vi "Scripting_ConvertBaseClassToSubClass.vi"(0 "BaseClass":refnum<vi>, 1 "NewBaseClass":path=path "C:/Documents and Settings/Micke/Skrivbord/My Computer/B_class/B.lvclass", 2 "SubClassTemplate":path=path "C:/Program/National Instruments/LabVIEW 8.2/resource/Framework/Providers/Endevo/ClassProviders/Provider_EndevoGOOP300/Templates/SubTemplate/SubTemplate.lvclass", 3 "GOOP4Style":bool, 5 "error in (no error)":errorcluster) -> (19 "error out":errorcluster={"status"=TRUE, "code"=1055, "source"="Property Node in Scripting_ConvertBaseClassToSubClass.vi"})   [LabVIEW 2012]
uses:
  <vilib>/Utility/miscctls.llb/LVPositionTypeDef.ctl
  <resource>/Framework/Providers/Open_GDS/ClassProviders/Provider_EndevoGOOP300/EndevoProviderName.ctl
  <resource>/Framework/Providers/Open_GDS/ClassProviders/Provider_EndevoGOOP300/Templates/EndevoTemplateNames.ctl
  <resource>/Framework/Providers/Open_GDS/ClassProviders/Provider_EndevoGOOP400/EndevoG4ProviderName.ctl
  <resource>/Framework/Providers/Open_GDS/ClassProviders/Provider_EndevoGOOP400/Templates/EndevoG4TemplateNames.ctl
  <resource>/Framework/Providers/Open_GDS/ClassProviders/Provider_LvNativeClass/ClassWriterNative_class/ClassWriterNative.lvclass
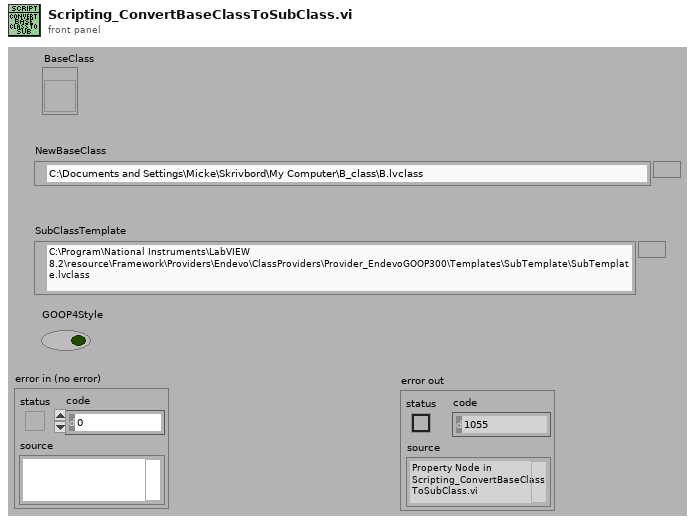
[diagram p1: front panel]
types:
  T1 = cluster{"NewBaseClass":refnum<vi>, "NewBaseCreate ":path, "NewBaseDestroy":path, "NewBaseKernel":path, "NewBaseAttribute":path, "NewBaseClassAttr":path, "NewBaseObjectRef":path, " BaseClass":refnum<vi>, "BaseCreate ":path, "BaseDestroy":path, "BaseKernel":path, "BaseAttribute":path, "BaseClassAttr":path, "BaseClassName":string, "BaseObjectRef":path, "AllBaseClassFiles":path[], "SubNewVi":path, "ObjectRef":refnum<vi>, "BaseNewVi":path, "BaseDeleteVi":path, "SubTemplateKernel":path, "ClassVIs":refnum<vi>[], "SubTemplateClass":refnum<vi>, "BaseTemplateClass":refnum<vi>, "BaseTemplateKernel":path, "BaseAttrRef":refnum<vi>, "BaseClassAttrRef":refnum<vi>, "KernelRef":refnum<vi>, "TemplateVersionUsed":string, "NewBaseNewVI":path, "Singleton":bool, "BaseGetInstance":path, "NewBaseGetInstance":path, "App":refnum<vi>}
  T2 = typedef "LVPositionTypeDef.ctl" = cluster{"Left":i32, "Top":i32}
  T3 = typedef "EndevoTemplateNames.ctl" = enum16{"BaseTemplate", "SubTemplate", "BaseTemplate_4x4x4", "SubTemplate_4x4x4", "SingletonTemplate"}
  T4 = typedef "EndevoProviderName.ctl" = enum16{"EndevoGOOP300"}
  T5 = typedef "EndevoG4TemplateNames.ctl" = enum16{"G4BaseTemplate_Simple_4x4x4", "G4SubTemplate_Simple_4x4x4", "G4BaseTemplate_Simple_6x8x6", "G4SubTemplate_Simple_6x8x6", "G4BaseTemplate_Singleton_4x4x4", "G4SubTemplate_Singleton_4x4x4", "G4BaseTemplate_Singleton_6x8x6", "G4SubTemplate_Singleton_6x8x6", "G4InterfaceTemplate_6x8x6", "G4InterfaceTemplate_4x4x4"}
  T6 = typedef "EndevoG4ProviderName.ctl" = enum16{"EndevoGOOP400"}
  T7 = cluster{"Major":u16, "Minor":u16, "Fix":u16, "Build":u16}
  T8 = cluster{i32, "WireTermSource":refnum<vi>, "AllWireTerminalDrains":refnum<vi>[]}[]
  T9 = cluster{i32, "AllWireTerminalDrains":refnum<vi>[]}[]
  T10 = typedef "GDSLvCLass_ClassSettingsType.ctl" = cluster{"ClassProviderName":string, "ClassTemplateUsed":string, "ClassTemplateVersion":string, "ClassDescription":string, "PlugIns":T11[], "ConnectorPanePattern":string}
  T11 = typedef "GDSLvClass_PlugIn.ctl" = cluster{"Type":T12, "ID":string, "Version":string, "Path":path, "Name":string, "Data":variant}
  T12 = typedef "GDSLvClass_PlugInTypes.ctl" = enum16{"DesignPattern", "MethodTypes"}
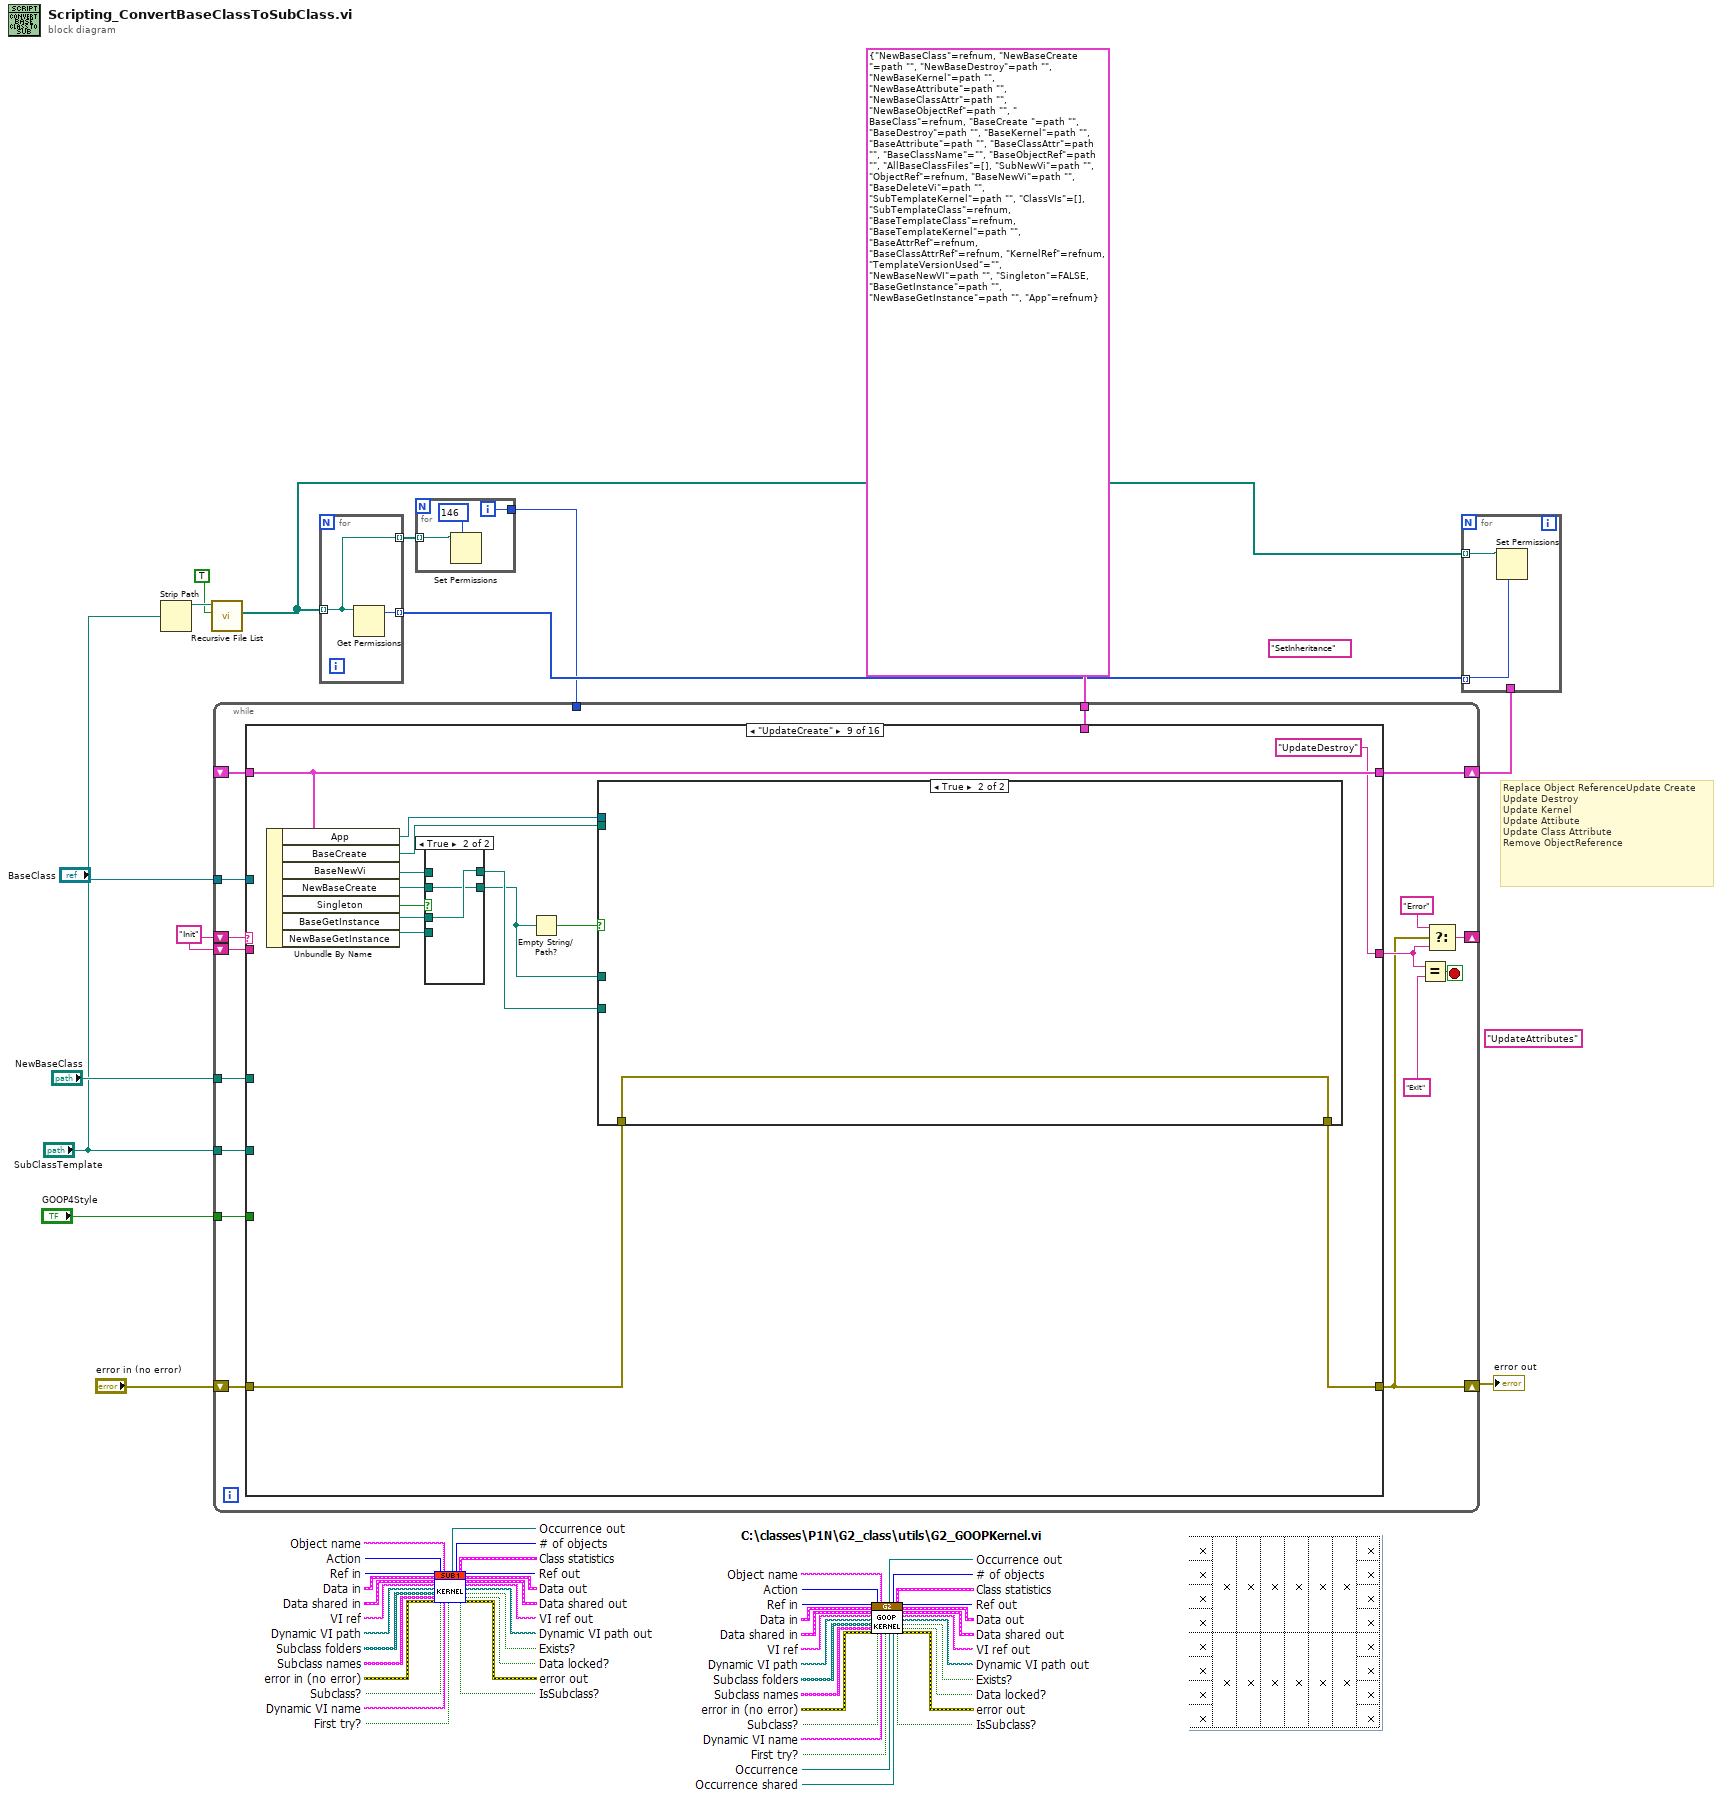
[diagram p0: block diagram]
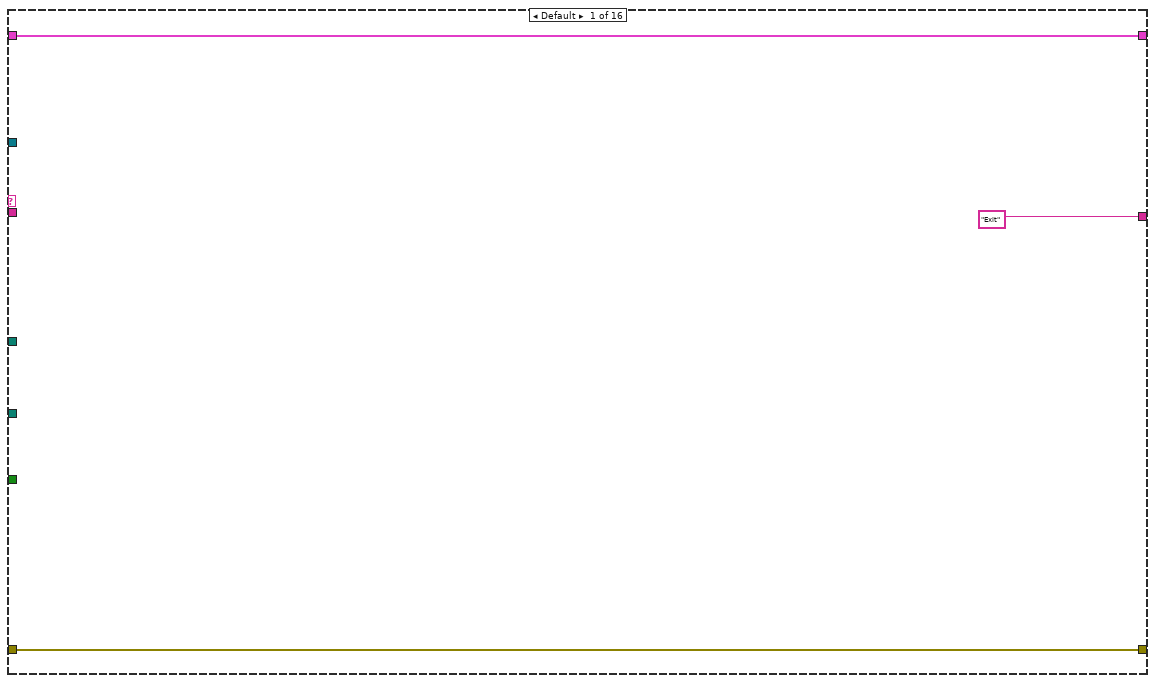
[diagram p2: hidden frame]
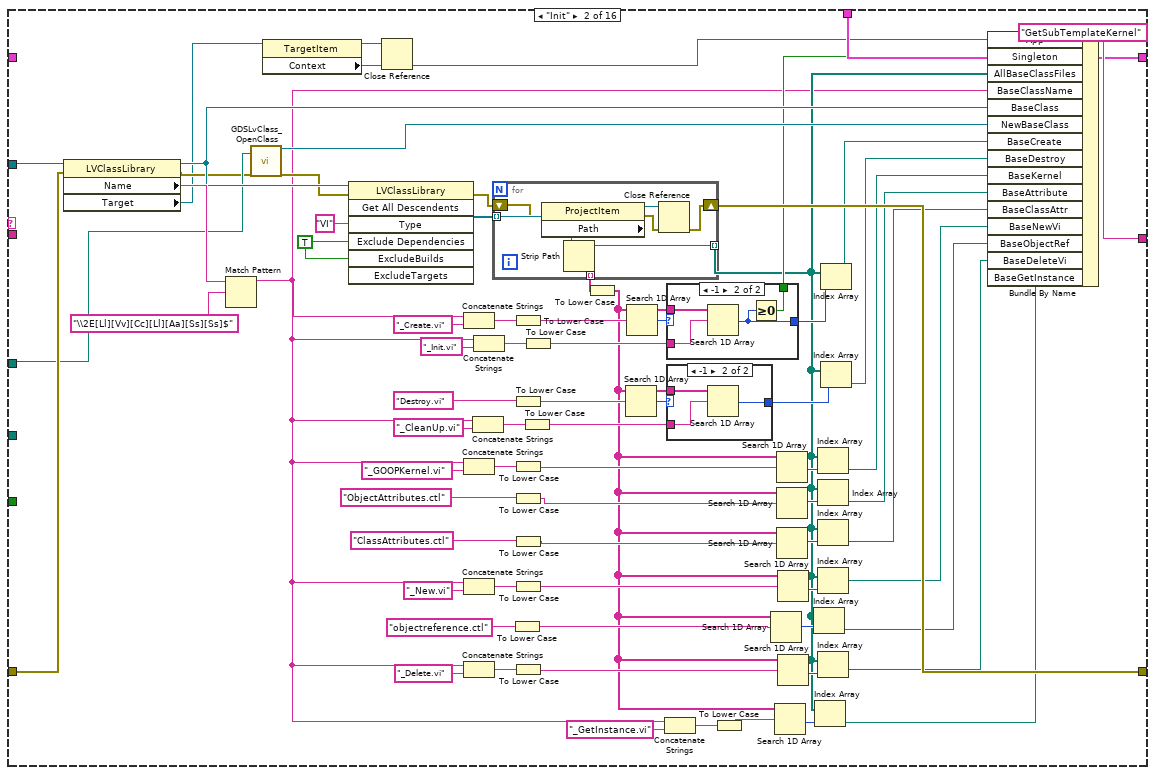
[diagram p3: hidden frame]
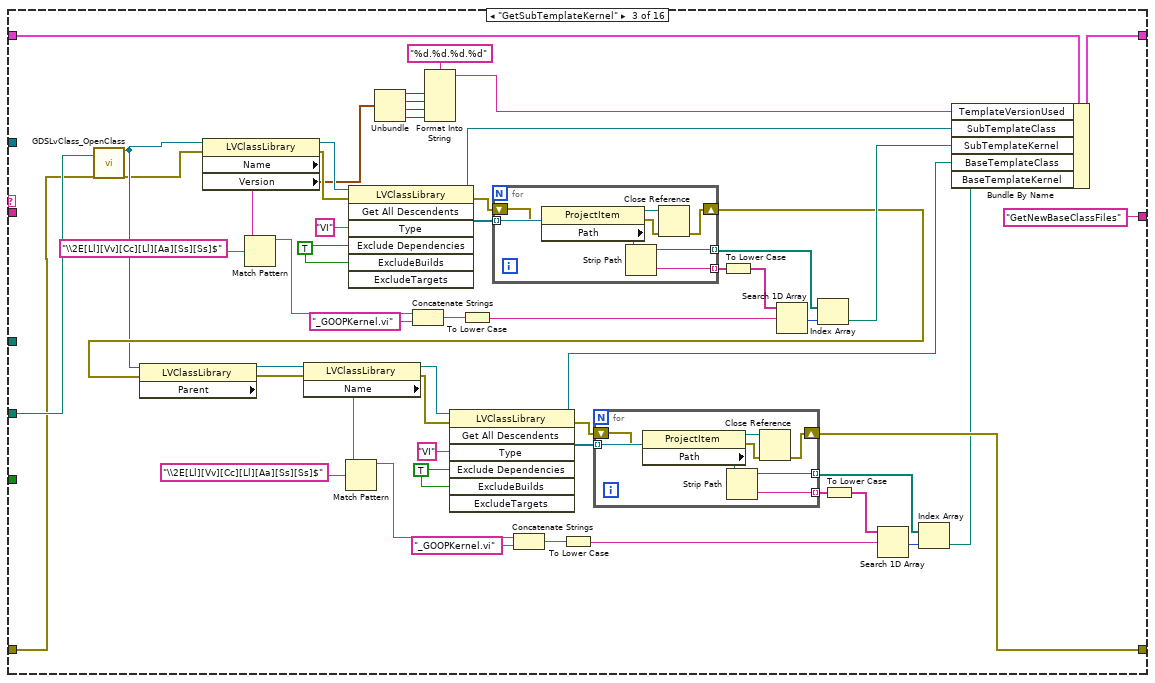
[diagram p6: hidden frame]
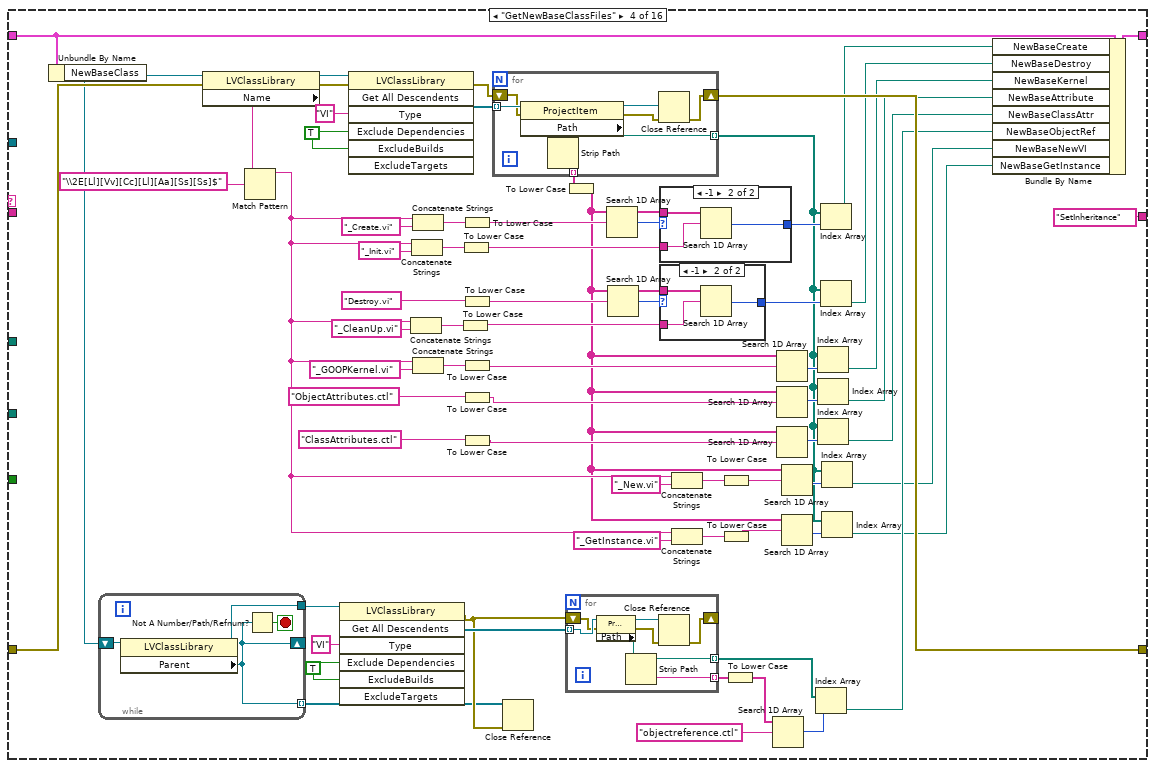
[diagram p7: hidden frame]
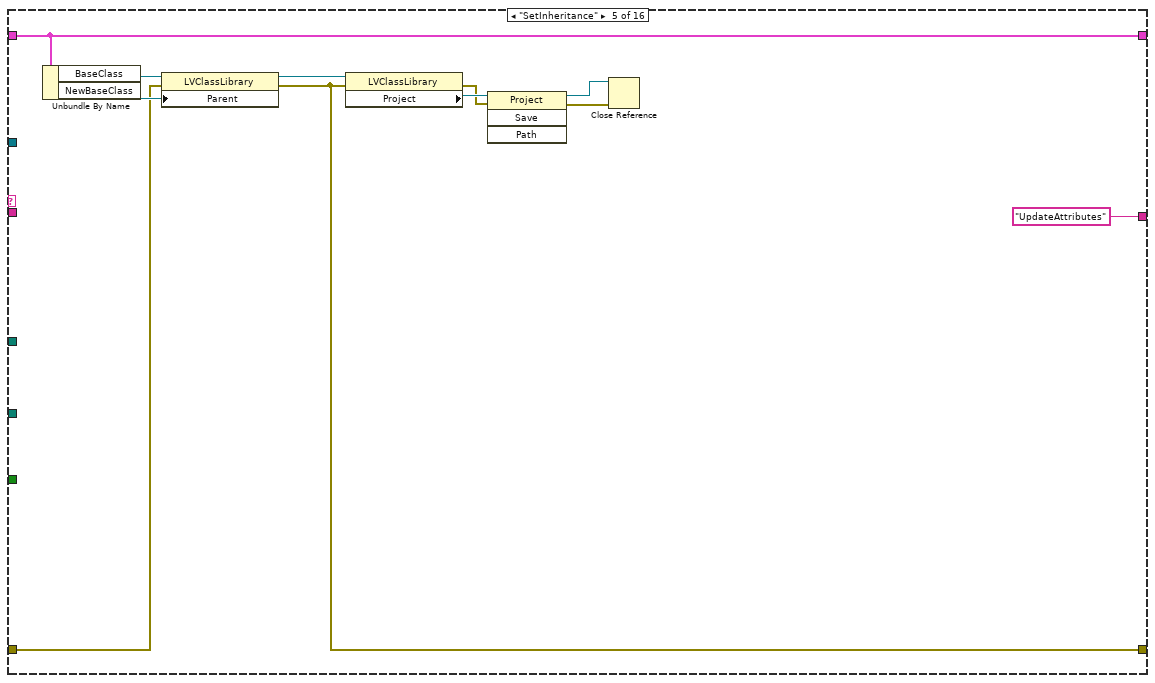
[diagram p10: hidden frame]
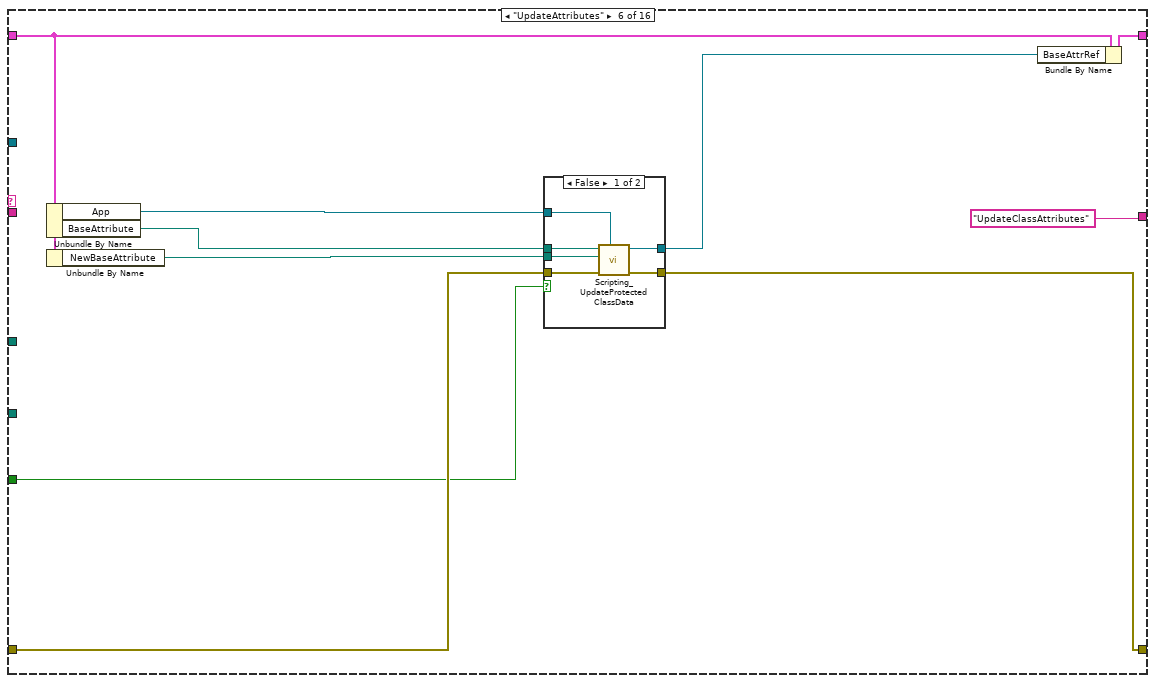
[diagram p11: hidden frame]
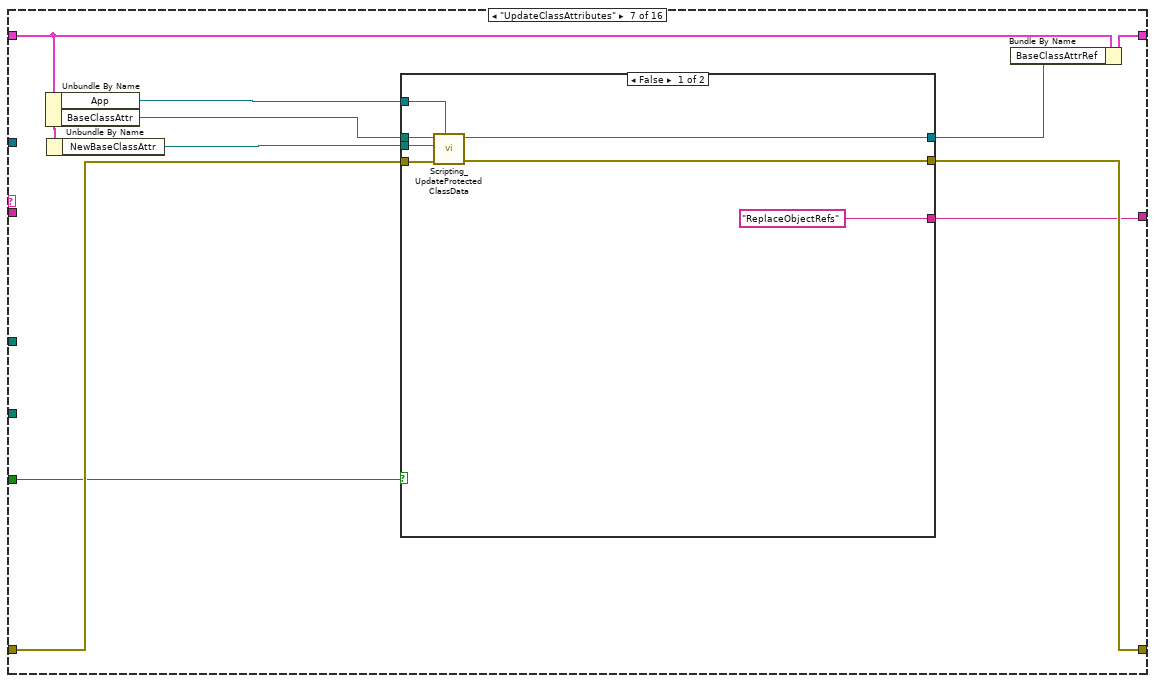
[diagram p13: hidden frame]
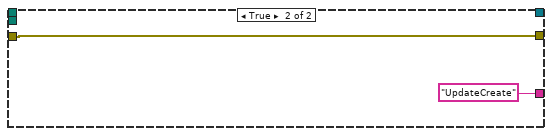
[diagram p14: hidden frame]
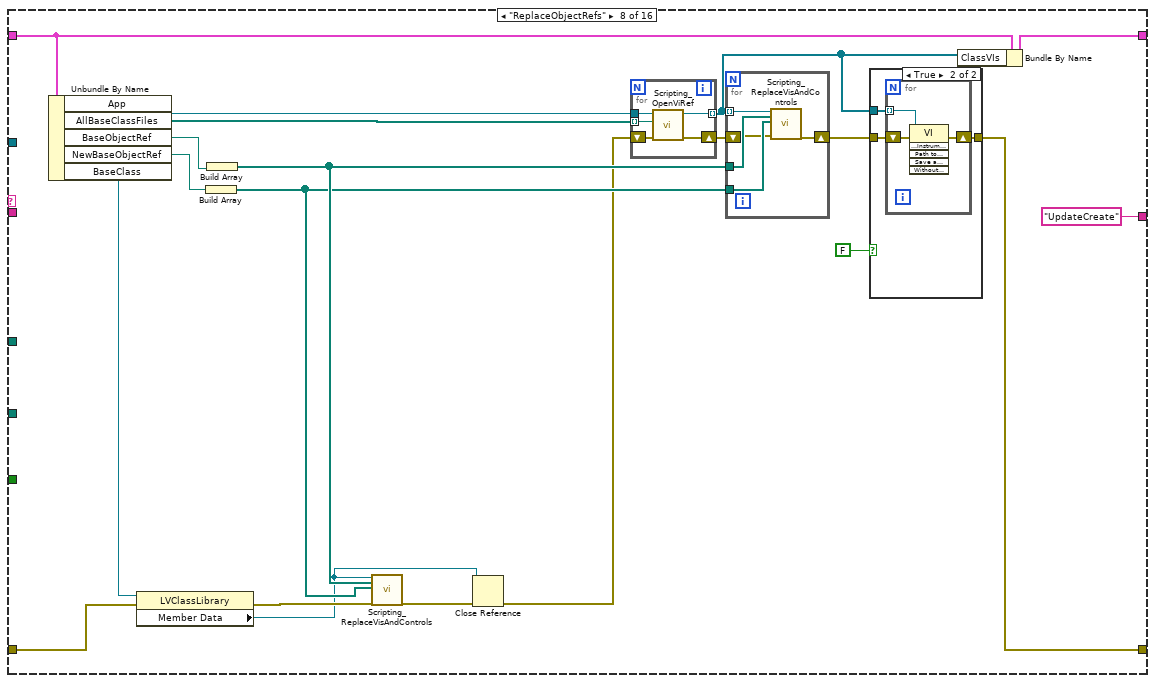
[diagram p15: hidden frame]
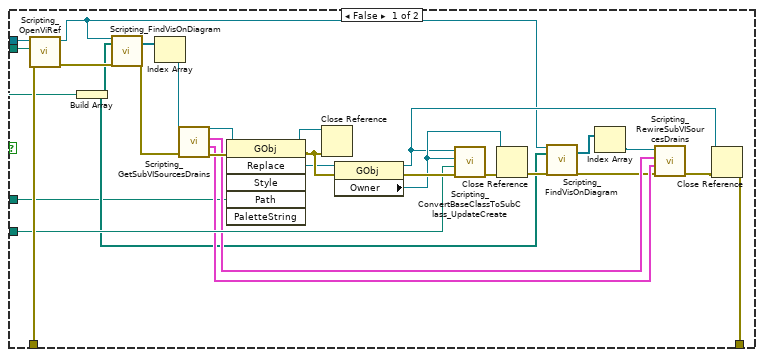
[diagram p17: hidden frame]
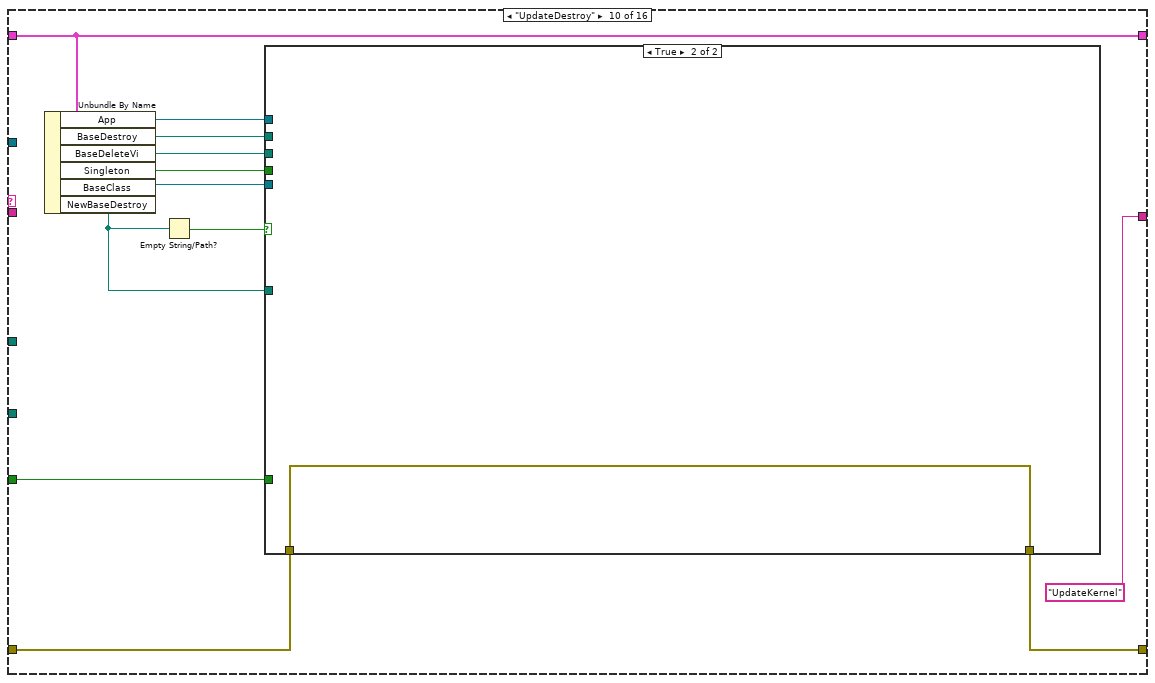
[diagram p19: hidden frame]
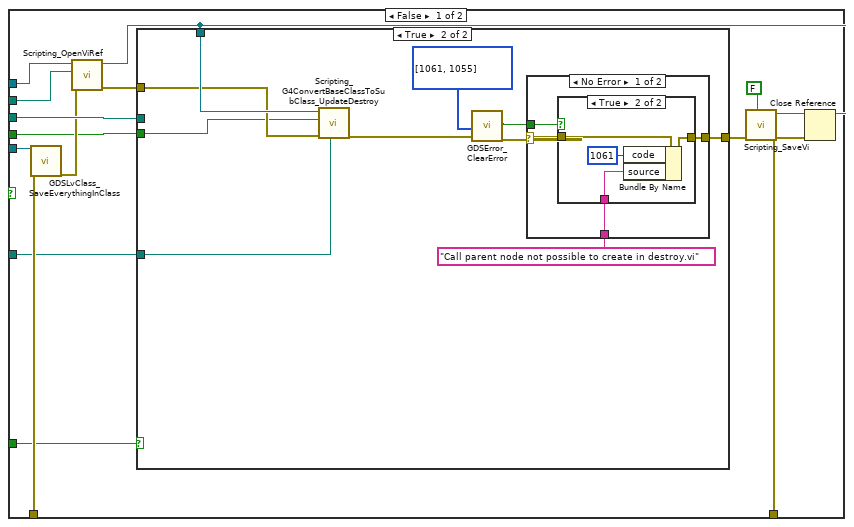
[diagram p20: hidden frame]
diagram:
  (unwired) "SetInheritance"
  (unwired) "UpdateAttributes"
  w10 = "Init"
  # "Replace Object ReferenceUpdate Create\nUpdate Destroy\nUpdate Kernel\nUpdate Attibute\nUpdate Class Attribute\nRemove ObjectReference"
  n1 = Strip Path(path="SubClassTemplate") -> (stripped path=w9:path)  [unwired: 1 out]
  n2 = call <vilib>:"Recursive File List.vi"("Treat LLBs as Folders?"=TRUE, "Folder Path"=w9) -> ("All Files in Dir"=w4:path[])  [unwired: 5 in, 4 out]
  n3 = for {
    tunnel: w4 -> [w16] mode=indexing
    tunnel: [w17] -> w6 mode=indexing
    tunnel: [w16] -> w3 mode=indexing
    n4 = Get Permissions(11:w16) -> (5:w17:i16)  [unwired: 1 in, 4 out]
  }
  n5 = for {
    tunnel: w3 -> [w20] mode=indexing
    tunnel: [w18] -> w5
    i -> [w18]
    n6 = Set Permissions(7:i16 146 ("permissions"), 11:w20) -> ()  [unwired: 3 in, 2 out]
  }
  n7 = while {
    shift-right: [w29] -> w14
    shift-left: "error in (no error)" -> [w36]
    shift-right: [w34] -> _
    shift-left: w10 -> [w35]
    shift-right: [w28] -> w7
    shift-left: _ -> [w27]
    tunnel: "BaseClass" -> [w26]
    tunnel: T1 {"NewBaseClass"=refnum, "NewBaseCreate "=path "", "NewBaseDestroy"=path "", "NewBaseKernel"=path "", "NewBaseAttribute"=path "", "NewBaseClassAttr"=path "", "NewBaseObjectRef"=path "", " BaseClass"=refnum, "BaseCreate "=path "", "BaseDestroy"=path "", "BaseKernel"=path "", "BaseAttribute"=path "", "BaseClassAttr"=path "", "BaseClassName"="", "BaseObjectRef"=path "", "AllBaseClassFiles"=[], "SubNewVi"=path "", "ObjectRef"=refnum, "BaseNewVi"=path "", "BaseDeleteVi"=path "", "SubTemplateKernel"=path "", "ClassVIs"=[], "SubTemplateClass"=refnum, "BaseTemplateClass"=refnum, "BaseTemplateKernel"=path "", "BaseAttrRef"=refnum, "BaseClassAttrRef"=refnum, "KernelRef"=refnum, "TemplateVersionUsed"="", "NewBaseNewVI"=path "", "Singleton"=FALSE, "BaseGetInstance"=path "", "NewBaseGetInstance"=path "", "App"=refnum} -> [w25]
    tunnel: "NewBaseClass" -> [w24]
    tunnel: "SubClassTemplate" -> [w23]
    shift-left: w10 -> [w22]
    tunnel: w5 -> [_]
    tunnel: "GOOP4Style" -> [w21]
    stop <- w33 stop-if-true
    n8 = case shown="\"UpdateCreate\"" w35 {
      tunnel: w36 -> [w39 w79 w139 w238 w301 w312 w327 w349 w389 w431 w505 w645 w675 w717 w762 w772]
      tunnel: [w39 w104 w143 w257 w294 w308 w326 w346 w388 w429 w504 w644 w674 w701 w761 w772] -> w29
      tunnel: ["Exit" "GetSubTemplateKernel" "GetNewBaseClassFiles" "SetInheritance" "UpdateAttributes" "UpdateClassAttributes" w323 "UpdateCreate" "UpdateDestroy" "UpdateKernel" w506 "UpdateClassInfo" "RemoveObjectRef_And_SaveFiles" "UpdateAllDerivedClasses" "CloseReferences" "Exit"] -> w30
      tunnel: [w37 w112 w183 w267 w303 w309 w330 w354 w391 w436 w502 w642 w672 w716 w764 w770] -> w28
      tunnel: w27 -> [w37 _ w171 w239 w303 w310 w331 w355 w391 w436 w503 w642 w672 w716 w764 w770]
      tunnel: w26 -> [_ w78 _ _ _ _ _ _ _ _ _ _ _ _ w760 _]
      tunnel: w25 -> [_ w86 _ _ _ _ _ _ _ _ _ _ _ _ _ _]
      tunnel: w24 -> [_ w66 _ _ _ _ _ _ _ _ _ _ _ _ _ _]
      tunnel: w23 -> [_ _ w168 _ _ _ _ _ _ _ _ _ _ _ _ _]
      tunnel: w22 -> [_ _ _ _ _ _ _ _ _ _ _ _ _ _ _ w771]
      tunnel: w21 -> [_ _ _ _ _ w306 w324 _ _ w430 w501 w646 w665 w699 w759 _]
      frame Default {
      }
      frame "Init" {
        w62 = TRUE ("ExcludeDependencies")
        n9 = property class="LVClassLibrary"(reference=w78, error in=w79) -> (reference out=w76:refnum<vi>, error out=w65:errorcluster, "Name"=w77:string, "Target"=w42:refnum<vi>)
        n10 = Match Pattern(string=w77, regular expression="\\2E[Ll][Vv][Cc][Ll][Aa][Ss][Ss]$") -> (before substring=w44:string)  [unwired: 1 in, 3 out]
        n11 = call <resource>:"GDSLvClass_OpenClass.vi"("ClassToOpen"=w66, "error in (no error)"=w65) -> ("LVClass.Open"=w63:refnum<vi>, "error out"=w64:errorcluster)  [unwired: 16 in]
        n12 = property class="TargetItem"(reference=w42) -> (reference out=w41:refnum<vi>, "Context"=w40:refnum<vi>)  [unwired: 1 in, 1 out]
        n13 = invoke class="LVClassLibrary" method="Get All Descendents"(reference=w76, error in=w64, "Type"="VI", "Exclude Dependencies"=w62, "ExcludeBuilds"=w62) -> (error out=w109:errorcluster, "All Descendents"=w110:refnum<vi>[])  [unwired: 2 in, 5 out]
        n14 = Close Reference(reference=w41) -> ()  [unwired: 1 in, 1 out]
        n15 = Concatenate Strings(w44, "_Create.vi" ("string")) -> (w106:string)
        n16 = Concatenate Strings(w44, "_GOOPKernel.vi" ("string")) -> (w100:string)
        n17 = Concatenate Strings(w44, "_New.vi" ("string")) -> (w83:string)
        n18 = Concatenate Strings(w44, "_Delete.vi" ("string")) -> (w70:string)
        n19 = Concatenate Strings(w44, "_CleanUp.vi" ("string")) -> (w60:string)
        n20 = Concatenate Strings(w44, "_Init.vi" ("string")) -> (w61:string)
        n21 = for {
          tunnel: w110 -> [w129] mode=indexing
          shift-right: [w125] -> w104
          shift-left: w109 -> [w126]
          tunnel: [w124] -> w46 mode=indexing
          tunnel: [w123] -> w107 mode=indexing
          n22 = property class="ProjectItem"(reference=w129, error in=w126) -> (reference out=w128:refnum<vi>, error out=w127:errorcluster, "Path"=w124:path)
          n23 = Strip Path(path=w124) -> (name=w123:string)  [unwired: 1 out]
          n24 = Close Reference(reference=w128, error in (no error)=w127) -> (error out=w125:errorcluster)
        }
        n25 = To Lower Case(string="objectreference.ctl" ("element")) -> (all lower case string=w74:string)
        n26 = To Lower Case(string=w106) -> (all lower case string=w105:string)
        n27 = To Lower Case(string="Destroy.vi") -> (all lower case string=w102:string)
        n28 = To Lower Case(string=w100) -> (all lower case string=w98:string)
        n29 = To Lower Case(string="ObjectAttributes.ctl") -> (all lower case string=w93:string)
        n30 = To Lower Case(string="ClassAttributes.ctl") -> (all lower case string=w90:string)
        n31 = To Lower Case(string=w83) -> (all lower case string=w84:string)
        n32 = To Lower Case(string=w70) -> (all lower case string=w68:string)
        n33 = To Lower Case(string=w60) -> (all lower case string=w58:string)
        n34 = To Lower Case(string=w61) -> (all lower case string=w59:string)
        n35 = To Lower Case(string=w107) -> (all lower case string=w45:string[])
        n36 = Search 1D Array(1D array=w45, element=w102) -> (index of element=w55:i32)  [unwired: 1 in]
        n37 = Search 1D Array(1D array=w45, element=w105) -> (index of element=w57:i32)  [unwired: 1 in]
        n38 = Concatenate Strings(w44, "_GetInstance.vi" ("string")) -> (w49:string)
        n39 = case shown="-1" w57 {
          selector: w57 -> [w118 _]
          tunnel: w45 -> [_ w122]
          tunnel: w59 -> [_ w121]
          tunnel: [w118 w120] -> w56
          tunnel: [_ w119] -> w51
          frame 0, Default {
          }
          frame -1 {
            n40 = Search 1D Array(1D array=w122, element=w121) -> (index of element=w120:i32)  [unwired: 1 in]
            n41 = Greater Or Equal To 0?(x=w120) -> (x >= 0?=w119:bool)
          }
        }
        n42 = case shown="-1" w55 {
          selector: w55 -> [w114 _]
          tunnel: w45 -> [_ w117]
          tunnel: w58 -> [_ w116]
          tunnel: [w114 w115] -> w54
          frame 0, Default {
          }
          frame -1 {
            n43 = Search 1D Array(1D array=w117, element=w116) -> (index of element=w115:i32)  [unwired: 1 in]
          }
        }
        n44 = To Lower Case(string=w49) -> (all lower case string=w47:string)
        n45 = Search 1D Array(1D array=w45, element=w74) -> (index of element=w75:i32)  [unwired: 1 in]
        n46 = Search 1D Array(1D array=w45, element=w47) -> (index of element=w48:i32)  [unwired: 1 in]
        n47 = Search 1D Array(1D array=w45, element=w98) -> (index of element=w97:i32)  [unwired: 1 in]
        n48 = Search 1D Array(1D array=w45, element=w93) -> (index of element=w92:i32)  [unwired: 1 in]
        n49 = Search 1D Array(1D array=w45, element=w90) -> (index of element=w91:i32)  [unwired: 1 in]
        n50 = Search 1D Array(1D array=w45, element=w84) -> (index of element=w81:i32)  [unwired: 1 in]
        n51 = Search 1D Array(1D array=w45, element=w68) -> (index of element=w69:i32)  [unwired: 1 in]
        n52 = Index Array(array=w46, index=w75) -> (element=w72:path)
        n53 = Index Array(array=w46, index=w48) -> (element=w43:path)
        n54 = Index Array(array=w46, index=w97) -> (element=w89:path)
        n55 = Index Array(array=w46, index=w92) -> (element=w88:path)
        n56 = Index Array(array=w46, index=w91) -> (element=w87:path)
        n57 = Index Array(array=w46, index=w81) -> (element=w80:path)
        n58 = Index Array(array=w46, index=w69) -> (element=w67:path)
        n59 = Index Array(array=w46, index=w56) -> (element=w101:path)
        n60 = Index Array(array=w46, index=w54) -> (element=w96:path)
        n61 = Bundle By Name(cluster=w86, "App"=w40, "Singleton"=w51, "AllBaseClassFiles"=w46, "BaseClassName"=w44, "BaseClass"=w76, "NewBaseClass"=w63, "BaseCreate"=w101, "BaseDestroy"=w96, "BaseKernel"=w89, "BaseAttribute"=w88, "BaseClassAttr"=w87, "BaseNewVi"=w80, "BaseObjectRef"=w72, "BaseDeleteVi"=w67, "BaseGetInstance"=w43) -> (w112:T1)
      }
      frame "GetSubTemplateKernel" {
        w137 = TRUE ("ExcludeDependencies")
        w138 = TRUE ("ExcludeDependencies")
        n62 = call <resource>:"GDSLvClass_OpenClass.vi"("ClassToOpen"=w168, "error in (no error)"=w139) -> ("LVClass.Open"=w161:refnum<vi>, "error out"=w140:errorcluster)  [unwired: 16 in]
        n63 = property class="LVClassLibrary"(reference=w161, error in=w140) -> (reference out=w178:refnum<vi>, error out=w179:errorcluster, "Name"=w170:string, "Version"=w131:T7)
        n64 = Match Pattern(string=w170, regular expression="\\2E[Ll][Vv][Cc][Ll][Aa][Ss][Ss]$") -> (before substring=w167:string)  [unwired: 1 in, 3 out]
        n65 = invoke class="LVClassLibrary" method="Get All Descendents"(reference=w178, error in=w179, "Type"="VI", "Exclude Dependencies"=w137, "ExcludeBuilds"=w137) -> (reference out=w163:refnum<vi>, error out=w180:errorcluster, "All Descendents"=w181:refnum<vi>[])  [unwired: 2 in, 4 out]
        n66 = Unbundle(w131) -> ("Major"=w136:u16, "Minor"=w135:u16, "Fix"=w134:u16, "Build"=w133:u16)
        n67 = Concatenate Strings(w167, "_GOOPKernel.vi" ("string")) -> (w176:string)
        n68 = Format Into String(format string="%d.%d.%d.%d", w136, w135, w134, w133) -> (resulting string=w130:string)  [unwired: 2 in, 1 out]
        n69 = To Lower Case(string=w176) -> (all lower case string=w174:string)
        n70 = for {
          tunnel: w181 -> [w197] mode=indexing
          shift-right: [w193] -> w162
          shift-left: w180 -> [w194]
          tunnel: [w192] -> w166 mode=indexing
          tunnel: [w191] -> w177 mode=indexing
          n71 = property class="ProjectItem"(reference=w197, error in=w194) -> (reference out=w196:refnum<vi>, error out=w195:errorcluster, "Path"=w192:path)
          n72 = Strip Path(path=w192) -> (name=w191:string)  [unwired: 1 out]
          n73 = Close Reference(reference=w196, error in (no error)=w195) -> (error out=w193:errorcluster)
        }
        n74 = property class="LVClassLibrary"(reference=w161, error in=w162) -> (error out=w145:errorcluster, "Parent"=w146:refnum<vi>)  [unwired: 1 out]
        n75 = property class="LVClassLibrary"(reference=w146, error in=w145) -> (reference out=w151:refnum<vi>, error out=w150:errorcluster, "Name"=w157:string)
        n76 = Match Pattern(string=w157, regular expression="\\2E[Ll][Vv][Cc][Ll][Aa][Ss][Ss]$") -> (before substring=w158:string)  [unwired: 1 in, 3 out]
        n77 = invoke class="LVClassLibrary" method="Get All Descendents"(reference=w151, error in=w150, "Type"="VI", "Exclude Dependencies"=w138, "ExcludeBuilds"=w138) -> (reference out=w144:refnum<vi>, error out=w149:errorcluster, "All Descendents"=w148:refnum<vi>[])  [unwired: 2 in, 4 out]
        n78 = Concatenate Strings(w158, "_GOOPKernel.vi" ("string")) -> (w153:string)
        n79 = To Lower Case(string=w153) -> (all lower case string=w155:string)
        n80 = for {
          tunnel: w148 -> [w190] mode=indexing
          shift-right: [w186] -> w143
          shift-left: w149 -> [w187]
          tunnel: [w185] -> w159 mode=indexing
          tunnel: [w184] -> w152 mode=indexing
          n81 = property class="ProjectItem"(reference=w190, error in=w187) -> (reference out=w189:refnum<vi>, error out=w188:errorcluster, "Path"=w185:path)
          n82 = Strip Path(path=w185) -> (name=w184:string)  [unwired: 1 out]
          n83 = Close Reference(reference=w189, error in (no error)=w188) -> (error out=w186:errorcluster)
        }
        n84 = To Lower Case(string=w177) -> (all lower case string=w165:string[])
        n85 = Search 1D Array(1D array=w165, element=w174) -> (index of element=w173:i32)  [unwired: 1 in]
        n86 = Index Array(array=w166, index=w173) -> (element=w172:path)
        n87 = To Lower Case(string=w152) -> (all lower case string=w160:string[])
        n88 = Search 1D Array(1D array=w160, element=w155) -> (index of element=w156:i32)  [unwired: 1 in]
        n89 = Index Array(array=w159, index=w156) -> (element=w142:path)
        n90 = Bundle By Name(cluster=w171, "TemplateVersionUsed"=w130, "SubTemplateClass"=w163, "SubTemplateKernel"=w172, "BaseTemplateClass"=w144, "BaseTemplateKernel"=w142) -> (w183:T1)
      }
      frame "GetNewBaseClassFiles" {
        w223 = TRUE ("ExcludeDependencies")
        w224 = TRUE ("ExcludeDependencies")
        n91 = Unbundle By Name(w239) -> ("NewBaseClass"=w236:refnum<vi>)
        n92 = while {
          shift-right: [w284] -> _
          shift-left: w236 -> [w285]
          tunnel: [w284] -> w206 mode=indexing
          tunnel: [w283] -> w234
          stop <- w286 stop-if-true
          n93 = property class="LVClassLibrary"(reference=w285) -> (reference out=w283:refnum<vi>, "Parent"=w284:refnum<vi>)  [unwired: 1 in, 1 out]
          n94 = Not A Number/Path/Refnum?(number/path/refnum=w284) -> (NaN/Path/Refnum?=w286:bool)
        }
        n95 = property class="LVClassLibrary"(reference=w236, error in=w238) -> (reference out=w262:refnum<vi>, error out=w263:errorcluster, "Name"=w237:string)
        n96 = Match Pattern(string=w237, regular expression="\\2E[Ll][Vv][Cc][Ll][Aa][Ss][Ss]$") -> (before substring=w203:string)  [unwired: 1 in, 3 out]
        n97 = invoke class="LVClassLibrary" method="Get All Descendents"(reference=w234, "Type"="VI", "Exclude Dependencies"=w224, "ExcludeBuilds"=w224) -> (error out=w207:errorcluster, "All Descendents"=w233:refnum<vi>[])  [unwired: 3 in, 5 out]
        n98 = invoke class="LVClassLibrary" method="Get All Descendents"(reference=w262, error in=w263, "Type"="VI", "Exclude Dependencies"=w223, "ExcludeBuilds"=w223) -> (error out=w264:errorcluster, "All Descendents"=w265:refnum<vi>[])  [unwired: 2 in, 5 out]
        n99 = Concatenate Strings(w203, "_CleanUp.vi" ("string")) -> (w212:string)
        n100 = Concatenate Strings(w203, "_Init.vi" ("string")) -> (w213:string)
        n101 = Concatenate Strings(w203, "_Create.vi" ("string")) -> (w259:string)
        n102 = Concatenate Strings(w203, "_GOOPKernel.vi" ("string")) -> (w253:string)
        n103 = To Lower Case(string=w212) -> (all lower case string=w208:string)
        n104 = To Lower Case(string=w213) -> (all lower case string=w209:string)
        n105 = To Lower Case(string=w259) -> (all lower case string=w258:string)
        n106 = To Lower Case(string="Destroy.vi") -> (all lower case string=w255:string)
        n107 = To Lower Case(string=w253) -> (all lower case string=w251:string)
        n108 = To Lower Case(string="ObjectAttributes.ctl") -> (all lower case string=w246:string)
        n109 = To Lower Case(string="ClassAttributes.ctl") -> (all lower case string=w243:string)
        n110 = for {
          tunnel: w265 -> [w293] mode=indexing
          shift-right: [w289] -> w257
          shift-left: w264 -> [w290]
          tunnel: [w288] -> w201 mode=indexing
          tunnel: [w287] -> w260 mode=indexing
          n111 = property class="ProjectItem"(reference=w293, error in=w290) -> (reference out=w292:refnum<vi>, error out=w291:errorcluster, "Path"=w288:path)
          n112 = Strip Path(path=w288) -> (name=w287:string)  [unwired: 1 out]
          n113 = Close Reference(reference=w292, error in (no error)=w291) -> (error out=w289:errorcluster)
        }
        n114 = Close Reference(reference=w206, error in (no error)=w207) -> ()  [unwired: 1 out]
        n115 = To Lower Case(string=w260) -> (all lower case string=w200:string[])
        n116 = for {
          tunnel: w233 -> [w282] mode=indexing
          shift-right: [w278] -> _
          shift-left: w207 -> [w279]
          tunnel: [w277] -> w228 mode=indexing
          tunnel: [w276] -> w232 mode=indexing
          n117 = property class="ProjectItem"(reference=w282, error in=w279) -> (reference out=w281:refnum<vi>, error out=w280:errorcluster, "Path"=w277:path)
          n118 = Strip Path(path=w277) -> (name=w276:string)  [unwired: 1 out]
          n119 = Close Reference(reference=w281, error in (no error)=w280) -> (error out=w278:errorcluster)
        }
        n120 = Search 1D Array(1D array=w200, element=w258) -> (index of element=w217:i32)  [unwired: 1 in]
        n121 = Search 1D Array(1D array=w200, element=w255) -> (index of element=w215:i32)  [unwired: 1 in]
        n122 = case shown="-1" w217 {
          selector: w217 -> [w272 _]
          tunnel: w200 -> [_ w275]
          tunnel: w209 -> [_ w274]
          tunnel: [w272 w273] -> w216
          frame 0, Default {
          }
          frame -1 {
            n123 = Search 1D Array(1D array=w275, element=w274) -> (index of element=w273:i32)  [unwired: 1 in]
          }
        }
        n124 = case shown="-1" w215 {
          selector: w215 -> [w268 _]
          tunnel: w200 -> [_ w271]
          tunnel: w208 -> [_ w270]
          tunnel: [w268 w269] -> w214
          frame 0, Default {
          }
          frame -1 {
            n125 = Search 1D Array(1D array=w271, element=w270) -> (index of element=w269:i32)  [unwired: 1 in]
          }
        }
        n126 = Concatenate Strings(w203, "_New.vi" ("string")) -> (w221:string)
        n127 = Concatenate Strings(w203, "_GetInstance.vi" ("string")) -> (w204:string)
        n128 = To Lower Case(string=w221) -> (all lower case string=w222:string)
        n129 = To Lower Case(string=w204) -> (all lower case string=w199:string)
        n130 = To Lower Case(string=w232) -> (all lower case string=w226:string[])
        n131 = Search 1D Array(1D array=w226, element="objectreference.ctl") -> (index of element=w229:i32)  [unwired: 1 in]
        n132 = Search 1D Array(1D array=w200, element=w251) -> (index of element=w250:i32)  [unwired: 1 in]
        n133 = Search 1D Array(1D array=w200, element=w246) -> (index of element=w245:i32)  [unwired: 1 in]
        n134 = Search 1D Array(1D array=w200, element=w243) -> (index of element=w244:i32)  [unwired: 1 in]
        n135 = Search 1D Array(1D array=w200, element=w222) -> (index of element=w219:i32)  [unwired: 1 in]
        n136 = Search 1D Array(1D array=w200, element=w199) -> (index of element=w202:i32)  [unwired: 1 in]
        n137 = Index Array(array=w228, index=w229) -> (element=w227:path)
        n138 = Index Array(array=w201, index=w250) -> (element=w242:path)
        n139 = Index Array(array=w201, index=w245) -> (element=w241:path)
        n140 = Index Array(array=w201, index=w244) -> (element=w240:path)
        n141 = Index Array(array=w201, index=w216) -> (element=w254:path)
        n142 = Index Array(array=w201, index=w214) -> (element=w249:path)
        n143 = Index Array(array=w201, index=w219) -> (element=w218:path)
        n144 = Index Array(array=w201, index=w202) -> (element=w198:path)
        n145 = Bundle By Name(cluster=w239, "NewBaseCreate"=w254, "NewBaseDestroy"=w249, "NewBaseKernel"=w242, "NewBaseAttribute"=w241, "NewBaseClassAttr"=w240, "NewBaseObjectRef"=w227, "NewBaseNewVI"=w218, "NewBaseGetInstance"=w198) -> (w267:T1)
      }
      frame "SetInheritance" {
        n146 = Unbundle By Name(w303) -> ("BaseClass"=w304:refnum<vi>, "NewBaseClass"=w302:refnum<vi>)
        n147 = property class="LVClassLibrary"(reference=w304, error in=w301, "Parent"=w302) -> (reference out=w299:refnum<vi>, error out=w294:errorcluster)
        n148 = property class="LVClassLibrary"(reference=w299, error in=w294) -> (error out=w295:errorcluster, "Project"=w298:refnum<vi>)  [unwired: 1 out]
        n149 = invoke class="Project" method="Save"(reference=w298, error in=w295) -> (reference out=w296:refnum<vi>, error out=w297:errorcluster)  [unwired: 2 in, 2 out]
        n150 = Close Reference(reference=w296, error in (no error)=w297) -> ()  [unwired: 1 out]
      }
      frame "UpdateAttributes" {
        n151 = Unbundle By Name(w310) -> ("App"=w305:refnum<vi>, "BaseAttribute"=w313:path)
        n152 = Unbundle By Name(w310) -> ("NewBaseAttribute"=w311:path)
        n153 = case shown="False" w306 {
          tunnel: w313 -> [w320 _]
          tunnel: w312 -> [w319 w321]
          tunnel: w311 -> [w318 _]
          tunnel: [w317 w321] -> w308
          tunnel: [w316 _] -> w307
          tunnel: w305 -> [w315 _]
          frame False {
            n154 = call <resource>:"Scripting_UpdateProtectedClassData.vi"("AppRef"=w315, "error in (no error)"=w319, "NewBaseAttribute"=w318, "BaseAttribute"=w320) -> ("error out"=w317:errorcluster, "BaseAttributeReference"=w316:refnum<vi>)  [unwired: 6 in]
          }
          frame True {
          }
        }
        n155 = Bundle By Name(cluster=w310, "BaseAttrRef"=w307) -> (w309:T1)
      }
      frame "UpdateClassAttributes" {
        n156 = Unbundle By Name(w331) -> ("App"=w322:refnum<vi>, "BaseClassAttr"=w329:path)
        n157 = Unbundle By Name(w331) -> ("NewBaseClassAttr"=w328:path)
        n158 = case shown="False" w324 {
          tunnel: w329 -> [w338 _]
          tunnel: w328 -> [w337 _]
          tunnel: w327 -> [w336 w340]
          tunnel: [w335 w340] -> w326
          tunnel: [w334 _] -> w325
          tunnel: ["ReplaceObjectRefs" "UpdateCreate"] -> w323
          tunnel: w322 -> [w332 _]
          frame False {
            n159 = call <resource>:"Scripting_UpdateProtectedClassData.vi"("AppRef"=w332, "error in (no error)"=w336, "NewBaseAttribute"=w337, "BaseAttribute"=w338) -> ("error out"=w335:errorcluster, "BaseAttributeReference"=w334:refnum<vi>)  [unwired: 6 in]
          }
          frame True {
          }
        }
        n160 = Bundle By Name(cluster=w331, "BaseClassAttrRef"=w325) -> (w330:T1)
      }
      frame "ReplaceObjectRefs" {
        n161 = Unbundle By Name(w355) -> ("App"=w341:refnum<vi>, "AllBaseClassFiles"=w352:path[], "BaseObjectRef"=w359:path, "NewBaseObjectRef"=w358:path, "BaseClass"=w350:refnum<vi>)
        n162 = property class="LVClassLibrary"(reference=w350, error in=w349) -> (error out=w348:errorcluster, "Member Data"=w345:refnum<vi>)  [unwired: 1 out]
        n163 = Build Array(w358) -> (w356:path[])
        n164 = Build Array(w359) -> (w357:path[])
        n165 = call <resource>:"Scripting_ReplaceVisAndControls.vi"("ViRef"=w345, "OldVIsAndControls"=w357, "NewVIsAndControls"=w356, "error in (no error)"=w348) -> ("error out"=w342:errorcluster)  [unwired: 14 in, 1 out]
        n166 = Close Reference(reference=w345, error in (no error)=w342) -> (error out=w347:errorcluster)
        n167 = for {
          shift-right: [w372] -> w344
          shift-left: w347 -> [w371]
          tunnel: w352 -> [w370] mode=indexing
          tunnel: [w369] -> w351 mode=indexing
          tunnel: w341 -> [w368]
          n168 = call <resource>:"Scripting_OpenViRef.vi"("error in"=w371, "ViPath/ViName"=w370, "AppRef"=w368) -> ("error out"=w372:errorcluster, "vi reference"=w369:refnum<vi>)  [unwired: 7 in]
        }
        n169 = for {
          shift-right: [w377] -> w353
          shift-left: w344 -> [w374]
          tunnel: w357 -> [w376]
          tunnel: w356 -> [w375]
          tunnel: w351 -> [w373] mode=indexing
          n170 = call <resource>:"Scripting_ReplaceVisAndControls.vi"("ViRef"=w373, "OldVIsAndControls"=w376, "NewVIsAndControls"=w375, "error in (no error)"=w374) -> ("error out"=w377:errorcluster)  [unwired: 14 in, 1 out]
        }
        n171 = case shown="True" FALSE {
          tunnel: w353 -> [w361 w364]
          tunnel: w351 -> [_ w363]
          tunnel: [w361 w362] -> w346
          frame False {
          }
          frame True {
            n172 = for {
              shift-right: [w366] -> w362
              shift-left: w364 -> [w367]
              tunnel: w363 -> [w365] mode=indexing
              n173 = invoke class="VI" method="Save.Instrument"(reference=w365, error in=w367) -> (error out=w366:errorcluster)  [unwired: 4 in, 5 out]
            }
          }
        }
        n174 = Bundle By Name(cluster=w355, "ClassVIs"=w351) -> (w354:T1)
      }
      frame "UpdateCreate" {
        n175 = Unbundle By Name(w391) -> ("App"=w381:refnum<vi>, "BaseCreate"=w390:path, "BaseNewVi"=w386:path, "NewBaseCreate"=w385:path, "Singleton"=w387:bool, "BaseGetInstance"=w383:path, "NewBaseGetInstance"=w382:path)
        n176 = case shown="True" w387 {
          tunnel: w386 -> [w422 _]
          tunnel: w385 -> [w421 w423]
          tunnel: [w422 w424] -> w384
          tunnel: [w421 w423] -> w380
          tunnel: w383 -> [_ w424]
          tunnel: w382 -> [_ _]
          frame False {
          }
          frame True {
          }
        }
        n177 = Empty String/Path?(string/path=w380) -> (empty?=w378:bool)
        n178 = case shown="True" w378 {
          tunnel: w390 -> [w419 _]
          tunnel: w389 -> [w418 w420]
          tunnel: [w409 w420] -> w388
          tunnel: w384 -> [w408 _]
          tunnel: w381 -> [w393 _]
          tunnel: w380 -> [w392 _]
          frame False {
            n179 = call <resource>:"Scripting_OpenViRef.vi"("error in"=w418, "ViPath/ViName"=w419, "AppRef"=w393) -> ("error out"=w417:errorcluster, "vi reference"=w398:refnum<vi>)  [unwired: 7 in]
            n180 = Build Array(w408) -> (w397:path[])
            n181 = call <resource>:"Scripting_FindVisOnDiagram.vi"("ViRef"=w398, "VIsToSerachFor/ViName"=w397, "error in (no error)"=w417) -> ("VisFound"=w416:refnum<vi>[], "error out"=w407:errorcluster)  [unwired: 15 in]
            n182 = Index Array(array=w416) -> (element=w406:refnum<vi>)  [unwired: 1 in]
            n183 = call <resource>:"Scripting_GetSubVISourcesDrains.vi"("error in (no error)"=w407, "SubVIIn"=w406) -> ("error out"=w405:errorcluster, "DrainsSources"=w401:T8, "SourceDrains"=w402:T9, "SubVIOut"=w404:refnum<vi>)  [unwired: 6 in]
            n184 = invoke class="GObj" method="Replace"(reference=w404, error in=w405, "Path"=w392) -> (reference out=w415:refnum<vi>, error out=w414:errorcluster, "Replace"=w413:refnum<vi>)  [unwired: 3 in, 3 out]
            n185 = Close Reference(reference=w415, error in (no error)=w414) -> ()  [unwired: 1 out]
            n186 = property class="GObj"(reference=w413, error in=w414) -> (reference out=w400:refnum<vi>, error out=w412:errorcluster, "Owner"=w411:refnum<vi>)
            n187 = call <resource>:"Scripting_ConvertBaseClassToSubClass_UpdateCreate.vi"("error in (no error)"=w412, "NewViPath"=w408, "Diagram"=w411, "NewBaseCreate"=w400) -> ("error out"=w410:errorcluster)  [unwired: 7 in]
            n188 = Close Reference(reference=w411, error in (no error)=w410) -> (error out=w399:errorcluster)
            n189 = call <resource>:"Scripting_FindVisOnDiagram.vi"("ViRef"=w398, "VIsToSerachFor/ViName"=w397, "error in (no error)"=w399) -> ("VisFound"=w394:refnum<vi>[], "error out"=w395:errorcluster)  [unwired: 15 in]
            n190 = Index Array(array=w394) -> (element=w396:refnum<vi>)  [unwired: 1 in]
            n191 = call <resource>:"Scripting_RewireSubVISourcesDrains.vi"("error in"=w395, "DrainsSources"=w401, "SourceDrains"=w402, "SubVIIn"=w396) -> ("error out"=w403:errorcluster)  [unwired: 7 in]
            n192 = Close Reference(reference=w400, error in (no error)=w403) -> (error out=w409:errorcluster)
          }
          frame True {
          }
        }
      }
      frame "UpdateDestroy" {
        n193 = Unbundle By Name(w436) -> ("App"=w427:refnum<vi>, "BaseDestroy"=w435:path, "BaseDeleteVi"=w434:path, "Singleton"=w428:bool, "BaseClass"=w432:refnum<vi>, "NewBaseDestroy"=w426:path)
        n194 = Empty String/Path?(string/path=w426) -> (empty?=w425:bool)
        n195 = case shown="True" w425 {
          tunnel: w435 -> [w451 _]
          tunnel: w434 -> [w449 _]
          tunnel: w432 -> [w446 _]
          tunnel: w431 -> [w445 w500]
          tunnel: w430 -> [w442 _]
          tunnel: [w441 w500] -> w429
          tunnel: w428 -> [w439 _]
          tunnel: w427 -> [w438 _]
          tunnel: w426 -> [w437 _]
          frame False {
            n196 = call <resource>:"GDSLvClass_SaveEverythingInClass.vi"("ClassRefIn"=w446, "error in"=w445) -> ("error out"=w443:errorcluster)  [unwired: 16 in, 1 out]
            n197 = call <resource>:"Scripting_OpenViRef.vi"("error in"=w443, "ViPath/ViName"=w451, "AppRef"=w438) -> ("error out"=w450:errorcluster, "vi reference"=w447:refnum<vi>)  [unwired: 7 in]
            n198 = case shown="True" w442 {
              tunnel: w450 -> [w469 w482]
              tunnel: w449 -> [w464 _]
              tunnel: w447 -> [w460 w483]
              tunnel: [w454 w485] -> w444
              tunnel: w437 -> [w453 w484]
              tunnel: w439 -> [_ w480]
              frame False {
                n199 = Build Array(w464) -> (w468:path[])
                n200 = call <resource>:"Scripting_FindVisOnDiagram.vi"("ViRef"=w460, "VIsToSerachFor/ViName"=w468, "error in (no error)"=w469) -> ("VisFound"=w467:refnum<vi>[], "error out"=w463:errorcluster)  [unwired: 15 in]
                n201 = Index Array(array=w467) -> (element=w461:refnum<vi>)  [unwired: 1 in]
                n202 = property class="GObj"(reference=w461, error in=w463) -> (reference out=w466:refnum<vi>, error out=w465:errorcluster, "Owner"=w452:refnum<vi>)
                n203 = call <resource>:"Scripting_ConvertBaseClassToSubClass_UpdateDestroy.vi"("BaseClassDestroyViPath"=w453, "error in (no error)"=w465, "Diagram"=w452, "DeleteViRef"=w466) -> ("error out"=w462:errorcluster)  [unwired: 7 in]
                n204 = Close Reference(reference=w452, error in (no error)=w462) -> (error out=w459:errorcluster)
                n205 = call <resource>:"GDSError_ClearError.vi"("codes"=i32[] [1061, 1055], "error in (no error)"=w459) -> ("Cleared?"=w456:bool, "error out"=w457:errorcluster)  [unwired: 16 in]
                n206 = case shown="No Error" w457 {
                  selector: w457 -> [w472 w479]
                  tunnel: w456 -> [w473 _]
                  tunnel: "Call parent node not possible to create in destroy.vi" ("source") -> [w471 _]
                  tunnel: [w470 w479] -> w454
                  frame No Error {
                    n207 = case shown="True" w473 {
                      tunnel: w472 -> [w474 w478]
                      tunnel: w471 -> [_ w476]
                      tunnel: [w474 w475] -> w470
                      frame False {
                      }
                      frame True {
                        n208 = Bundle By Name(cluster=w478, "code"=1061, "source"=w476) -> (w475:errorcluster)
                      }
                    }
                  }
                  frame Error {
                  }
                }
              }
              frame True {
                n209 = call <resource>:"Scripting_G4ConvertBaseClassToSubClass_UpdateDestroy.vi"("BaseClassDestroyViPath"=w484, "error in (no error)"=w482, "Singleton"=w480, "ViRef"=w483) -> ("error out"=w481:errorcluster)  [unwired: 7 in]
                n210 = call <resource>:"GDSError_ClearError.vi"("codes"=i32[] [1061, 1055], "error in (no error)"=w481) -> ("Cleared?"=w487:bool, "error out"=w488:errorcluster)  [unwired: 16 in]
                n211 = case shown="No Error" w488 {
                  selector: w488 -> [w492 w499]
                  tunnel: w487 -> [w493 _]
                  tunnel: "Call parent node not possible to create in destroy.vi" ("source") -> [w491 _]
                  tunnel: [w490 w499] -> w485
                  frame No Error {
                    n212 = case shown="True" w493 {
                      tunnel: w492 -> [w494 w498]
                      tunnel: w491 -> [_ w496]
                      tunnel: [w494 w495] -> w490
                      frame False {
                      }
                      frame True {
                        n213 = Bundle By Name(cluster=w498, "code"=1061, "source"=w496) -> (w495:errorcluster)
                      }
                    }
                  }
                  frame Error {
                  }
                }
              }
            }
            n214 = call <resource>:"Scripting_SaveVi.vi"("ForceResaving(False)"=FALSE, "error in (no error)"=w444, "VIRefToSaveIn"=w447) -> ("error out"=w441:errorcluster, "VIRefToSaveOut"=w440:refnum<vi>)  [unwired: 7 in]
            n215 = Close Reference(reference=w440, error in (no error)=w441) -> ()  [unwired: 1 out]
          }
          frame True {
          }
        }
      }
      frame "UpdateKernel" {
        n216 = case shown="False" w501 {
          tunnel: ["UpdateClassInfo" "UpdateNEWVI"] -> w506
          tunnel: w505 -> [w560 w626]
          tunnel: [w512 w627] -> w504
          tunnel: w503 -> [w508 w625]
          tunnel: [w530 w624] -> w502
          frame False {
            n217 = Unbundle By Name(w508) -> ("App"=w507:refnum<vi>, "BaseKernel"=w581:path, "SubTemplateKernel"=w527:path)
            n218 = call <resource>:"Scripting_OpenViRef.vi"("error in"=w560, "ViPath/ViName"=w581, "AppRef"=w507) -> ("error out"=w580:errorcluster, "vi reference"=w571:refnum<vi>)  [unwired: 7 in]
            n219 = property class="VI"(reference=w571, error in=w580) -> (reference out=w566:refnum<vi>, error out=w529:errorcluster, "Diagram"=w569:refnum<vi>)
            n220 = Unbundle By Name(w508) -> ("SubTemplateClass"=w515:refnum<vi>, "BaseClass"=w514:refnum<vi>)
            n221 = property class="TopLvlDiag"(reference=w569, error in=w529) -> (reference out=w563:refnum<vi>, error out=w568:errorcluster, "AllObjs[]"=w567:refnum<vi>[])
            n222 = Unbundle By Name(w508) -> ("BaseAttribute"=w548:path, "BaseClassAttr"=w543:path, "BaseTemplateKernel"=w535:path, "NewBaseKernel"=w533:path)
            n223 = for {
              tunnel: w568 -> [w616]
              tunnel: w567 -> [w617] mode=indexing
              tunnel: [w616] -> w565
              n224 = invoke class="GObj" method="Delete"(reference=w617, error in=w616) -> (reference out=w618:refnum<vi>)  [unwired: 1 in, 2 out]
              n225 = Close Reference(reference=w618) -> ()  [unwired: 1 in, 1 out]
            }
            n226 = invoke class="VI" method="BD.Remove Bad Wires"(reference=w566, error in=w565) -> (reference out=w562:refnum<vi>, error out=w528:errorcluster)  [unwired: 1 in, 1 out]
            n227 = call <resource>:"Scripting_OpenViRef.vi"("error in"=w528, "ViPath/ViName"=w527, "AppRef"=w507) -> ("error out"=w525:errorcluster, "vi reference"=w524:refnum<vi>)  [unwired: 7 in]
            n228 = invoke class="VI" method="Fake Exec State"(reference=w524, "state"=2 ("State")) -> (reference out=w523:refnum<vi>)  [unwired: 2 in, 3 out]
            n229 = property class="VI"(reference=w523, error in=w525) -> (reference out=w520:refnum<vi>, error out=w579:errorcluster, "Diagram"=w576:refnum<vi>)
            n230 = invoke class="TopLvlDiag" method="Select All"(reference=w576, error in=w579) -> (reference out=w577:refnum<vi>, error out=w578:errorcluster)  [unwired: 1 in, 1 out]
            n231 = invoke class="TopLvlDiag" method="Copy Selection"(reference=w577, error in=w578) -> (reference out=w521:refnum<vi>, error out=w564:errorcluster)  [unwired: 1 in, 1 out]
            n232 = invoke class="TopLvlDiag" method="Paste"(reference=w563, error in=w564, "Pos"=T2 {"Left"=50, "Top"=50} ("Position")) -> (reference out=w541:refnum<vi>, error out=w542:errorcluster)  [unwired: 1 in, 2 out]
            n233 = invoke class="App" method="Clipboard.Empty"(error in=w542) -> (error out=w522:errorcluster)  [unwired: 2 in, 2 out]
            n234 = property class="VI"(reference=w562, error in=w522) -> (error out=w573:errorcluster, "Panel"=w574:refnum<vi>)  [unwired: 1 out]
            n235 = Close Reference(reference=w541) -> ()  [unwired: 1 in, 1 out]
            n236 = property class="Pnl"(reference=w574, error in=w573) -> (reference out=w540:refnum<vi>, error out=w572:errorcluster, "Controls[]"=w538:refnum<vi>[])
            n237 = Build Array(w533) -> (w532:path[])
            n238 = Build Array(w535) -> (w534:path[])
            n239 = Close Reference(reference=w521, error in (no error)=w522) -> (error out=w539:errorcluster)
            n240 = Close Reference(reference=w520, error in (no error)=w539) -> ()  [unwired: 1 out]
            n241 = for {
              tunnel: w538 -> [w619] mode=indexing
              shift-right: [w621] -> w570
              shift-left: w572 -> [w622]
              tunnel: [w620] -> w516 mode=indexing
              n242 = property class="Ctl"(reference=w619, error in=w622) -> (error out=w621:errorcluster, "Label.Text"=w620:string)  [unwired: 1 out]
            }
            n243 = property class="VI"(reference=w571, error in=w570) -> (reference out=w509:refnum<vi>, error out=w561:errorcluster, "ConPane"=w536:refnum<vi>)
            n244 = Search 1D Array(1D array=w516, element="Dynamic VI path" ("Id")) -> (index of element=w510:i32)  [unwired: 1 in]
            n245 = case shown="Default" w510 {
              tunnel: [string[] ["Data in", "Data out", "Action", "Ref in", "Ref out", "Data locked?", "error out", "error in (no error)", "Subclass?", "Object name", "Exists?", "Data shared out", "Data shared in", "Subclass names", "Class name", "Probe in", "Class statistics", "IsSubclass?", "Misc", "# of objects", "Occurrence out", "Occurrence", "Occurrence shared", "Probe out"] ("Array") string[] ["Data in", "Data out", "Action", "Ref in", "Ref out", "Data locked?", "error out", "error in (no error)", "Subclass?", "Object name", "Exists?", "Data shared out", "Data shared in", "Subclass folders", "Subclass names", "Dynamic VI name", "VI ref out", "Dynamic VI path", "Dynamic VI path out", "VI ref", "Class statistics", "IsSubclass?", "First try?", "# of objects", "Occurrence out", "Occurrence", "Occurrence shared"] ("Array")] -> w519
              tunnel: [i32[] [1, 21, 8, 0, 20, 26, 27, 7, 9, 10, 25, 22, 2, 6, 11, 3, 18, 19, 13, 16, 14, 15, 17, 23] i32[] [1, 21, 8, 0, 20, 26, 27, 7, 9, 10, 25, 22, 2, 5, 6, 11, 23, 4, 24, 3, 18, 19, 13, 16, 14, 15, 17]] -> w518
              frame -1 {
              }
              frame Default {
              }
            }
            n246 = for {
              tunnel: w516 -> [w606] mode=indexing
              tunnel: w536 -> [w615]
              tunnel: w519 -> [w608]
              tunnel: w538 -> [w609] mode=indexing
              tunnel: w518 -> [w613]
              shift-right: [w610] -> w537
              shift-left: w561 -> [w611]
              n247 = Search and Replace String(replace all?=TRUE ("replace all? (F)"), input string=w606, search string="\n", replace string=" " ("replace string (\"\")")) -> (result string=w605:string)  [unwired: 4 in, 3 out]
              n248 = Search 1D Array(1D array=w608, element=w605) -> (index of element=w614:i32)  [unwired: 1 in]
              n249 = Index Array(array=w613, index=w614) -> (element=w612:i32)
              n250 = invoke class="ConPane" method="AssignCtrlToTerm"(reference=w615, error in=w611, "Control"=w609, "TermIdx"=w612) -> (error out=w610:errorcluster)  [unwired: 1 in, 4 out]
            }
            n251 = Close Reference(reference=w536, error in (no error)=w537) -> ()  [unwired: 1 out]
            n252 = Search 1D Array(1D array=w516, element="Data in" ("Label.Text")) -> (index of element=w559:i32)  [unwired: 1 in]
            n253 = Search 1D Array(1D array=w516, element="Data out" ("Label.Text")) -> (index of element=w555:i32)  [unwired: 1 in]
            n254 = Search 1D Array(1D array=w516, element="Data shared in" ("Label.Text")) -> (index of element=w554:i32)  [unwired: 1 in]
            n255 = Search 1D Array(1D array=w516, element="Data shared out" ("Label.Text")) -> (index of element=w553:i32)  [unwired: 1 in]
            n256 = Index Array(array=w538, index=w559) -> (element=w557:refnum<vi>)
            n257 = Index Array(array=w538, index=w555) -> (element=w549:refnum<vi>)
            n258 = Index Array(array=w538, index=w554) -> (element=w545:refnum<vi>)
            n259 = Index Array(array=w538, index=w553) -> (element=w544:refnum<vi>)
            n260 = invoke class="Ctl" method="Replace"(reference=w557, error in=w537, "Path"=w548) -> (error out=w556:errorcluster)  [unwired: 3 in, 5 out]
            n261 = invoke class="Ctl" method="Replace"(reference=w549, error in=w556, "Path"=w548) -> (error out=w546:errorcluster)  [unwired: 3 in, 5 out]
            n262 = Close Reference(reference=w540) -> ()  [unwired: 1 in, 1 out]
            n263 = invoke class="Ctl" method="Replace"(reference=w545, error in=w546, "Path"=w543) -> (error out=w547:errorcluster)  [unwired: 3 in, 5 out]
            n264 = Bundle By Name(cluster=w508, "KernelRef"=w509) -> (w530:T1)
            n265 = invoke class="Ctl" method="Replace"(reference=w544, error in=w547, "Path"=w543) -> (error out=w511:errorcluster)  [unwired: 3 in, 5 out]
            n266 = case shown="-1" w510 {
              tunnel: w509 -> [_ w596]
              tunnel: w511 -> [w583 w595]
              tunnel: [w583 w594] -> w513
              tunnel: w515 -> [_ w591]
              tunnel: w514 -> [_ w590]
              frame Default {
              }
              frame -1 {
                n267 = property class="LVClassLibrary"(reference=w591) -> ("Path"=w587:path)  [unwired: 1 in, 2 out]
                n268 = property class="LVClassLibrary"(reference=w590) -> ("Path"=w589:path)  [unwired: 1 in, 2 out]
                n269 = call <vilib>:"Get File Extension.vi"("file"=w587) -> ("filename without extension"=w586:string)  [unwired: 7 in, 3 out]
                n270 = Concatenate Strings(w586, ".ctl" ("string")) -> (w585:string)
                n271 = Build Path(base path=w587, name or relative path=w585) -> (appended path=w588:path)
                n272 = Build Array(w588) -> (w593:path[])
                n273 = Build Array(w589) -> (w592:path[])
                n274 = call <resource>:"Scripting_ReplaceVisAndControls.vi"("ViRef"=w596, "OldVIsAndControls"=w593, "NewVIsAndControls"=w592, "error in (no error)"=w595) -> ("error out"=w594:errorcluster)  [unwired: 14 in, 1 out]
              }
            }
            n275 = call <resource>:"Scripting_ReplaceVisAndControls.vi"("ViRef"=w509, "OldVIsAndControls"=w534, "NewVIsAndControls"=w532, "error in (no error)"=w513) -> ("error out"=w531:errorcluster)  [unwired: 14 in, 1 out]
            n276 = for {
              tunnel: w538 -> [w602] mode=indexing
              shift-right: [w601] -> w512
              shift-left: w531 -> [w601]
              n277 = Close Reference(reference=w602, error in (no error)=w601) -> ()  [unwired: 1 out]
            }
          }
          frame True {
            n278 = disable-structure shown="Enabled" {
              disable-tunnel: [w636 w637] -> w627
              disable-tunnel: w626 -> [w634 w637]
              disable-tunnel: w625 -> [w631 w638]
              disable-tunnel: [w629 w638] -> w624
              frame Disabled {
                n279 = Unbundle By Name(w631) -> ("BaseKernel"=w635:path, "SubTemplateKernel"=w633:path)
                n280 = call <resource>:"Scripting_OpenViRef.vi"("error in"=w634, "ViPath/ViName"=w635) -> ("error out"=w632:errorcluster, "vi reference"=w630:refnum<vi>)  [unwired: 8 in]
                n281 = call <resource>:"Scripting_UpdateViFromTemplate.vi"("ViRef"=w630, "TemplateVI(Path or Ref)"=w633, "error in (no error)"=w632) -> ("TemplateVersionUsed"=w628:string, "error out"=w636:errorcluster)  [unwired: 15 in]
                n282 = Bundle By Name(cluster=w631, "KernelRef"=w630, "TemplateVersionUsed"=w628) -> (w629:T1)
              }
              frame Enabled {
              }
            }
          }
        }
      }
      frame "UpdateNEWVI" {
        n283 = Unbundle By Name(w642) -> ("App"=w641:refnum<vi>, "BaseNewVi"=w647:path, "NewBaseNewVI"=w640:path)
        n284 = Empty String/Path?(string/path=w640) -> (empty?=w639:bool)
        n285 = case shown="True" w639 {
          tunnel: w647 -> [w653 _]
          tunnel: w646 -> [w652 _]
          tunnel: w645 -> [w651 w660]
          tunnel: [w650 w660] -> w644
          tunnel: w641 -> [w649 _]
          tunnel: w640 -> [w648 _]
          frame False {
            n286 = case shown="True" w652 {
              tunnel: w651 -> [w654 w659]
              tunnel: [w654 w658] -> w650
              tunnel: w653 -> [_ w657]
              tunnel: w648 -> [_ w656]
              tunnel: w649 -> [_ w655]
              frame False {
              }
              frame True {
                n287 = call <resource>:"Scripting_UpdateNewVI.vi"("NewVI Ref or Path"=w657, "BaseClassNewVI Ref or Path(If empty the No base class will be used)"=w656, "error in (no error)"=w659, "AppRef"=w655) -> ("error out"=w658:errorcluster)  [unwired: 15 in]
              }
            }
          }
          frame True {
          }
        }
      }
      frame "UpdateClassInfo" {
        n288 = Unbundle By Name(w672) -> ("TemplateVersionUsed"=w668:string, "BaseClass"=w676:refnum<vi>)
        n289 = property class="LVClassLibrary"(reference=w676, error in=w675) -> (reference out=w671:refnum<vi>, error out=w670:errorcluster, "Description"=w677:string)
        n290 = call <resource>:"GDSLvClass_ReadClassType.vi"("Class Refnum In"=w671, "error in (no error)"=w670) -> ("Class Refnum Out"=w661:refnum<vi>, "ClassSettings"=w664:T10, "error out"=w669:errorcluster)  [unwired: 15 in]
        n291 = Unbundle By Name(w664) -> ("ClassTemplateUsed"=w663:string)
        n292 = call <resource>:"GOOP_ClassTemplateSplit.vi"("ClassItemRefIn"=w661, "FullClassTemplate"=w663) -> ("StandardTemplate"=w662:string)  [unwired: 12 in, 1 out]
        n293 = case shown="True" w665 {
          tunnel: [w681 w689] -> w667
          tunnel: [w680 w688] -> w666
          tunnel: w662 -> [w679 w691]
          frame False {
            n294 = Scan From String(input string=w679, default 1=EndevoTemplateNames."BaseTemplate" ("TemplateNames")) -> (output 1=w684:T3)  [unwired: 3 in, 3 out]
            n295 = case shown="\"BaseTemplate_4x4x4\"" w684 {
              tunnel: [EndevoTemplateNames."SubTemplate" ("TemplateNames") EndevoTemplateNames."SubTemplate_4x4x4" ("TemplateNames")] -> w683
              frame "BaseTemplate", Default {
              }
              frame "BaseTemplate_4x4x4" {
              }
            }
            n296 = Format Into String(EndevoProviderName."EndevoGOOP300" ("ProviderName")) -> (resulting string=w681:string)  [unwired: 3 in, 1 out]
            n297 = Format Into String(w683) -> (resulting string=w680:string)  [unwired: 3 in, 1 out]
          }
          frame True {
            n298 = Scan From String(input string=w691, default 1=EndevoG4TemplateNames."G4SubTemplate_Simple_4x4x4" ("TemplateNames")) -> (output 1=w693:T5)  [unwired: 3 in, 3 out]
            n299 = case shown="\"G4BaseTemplate_Singleton_6x8x6\"" w693 {
              tunnel: [EndevoG4TemplateNames."G4SubTemplate_Simple_4x4x4" ("TemplateNames") EndevoG4TemplateNames."G4SubTemplate_Simple_6x8x6" ("TemplateNames") EndevoG4TemplateNames."G4SubTemplate_Singleton_4x4x4" ("TemplateNames") EndevoG4TemplateNames."G4SubTemplate_Singleton_6x8x6" ("TemplateNames")] -> w694
              frame "G4BaseTemplate_Simple_4x4x4", Default {
              }
              frame "G4BaseTemplate_Simple_6x8x6" {
              }
              frame "G4BaseTemplate_Singleton_4x4x4" {
              }
              frame "G4BaseTemplate_Singleton_6x8x6" {
              }
            }
            n300 = Format Into String(EndevoG4ProviderName."EndevoGOOP400" ("ProviderName")) -> (resulting string=w689:string)  [unwired: 3 in, 1 out]
            n301 = Format Into String(w694) -> (resulting string=w688:string)  [unwired: 3 in, 1 out]
          }
        }
        n302 = Bundle By Name(cluster=w664, "ClassTemplateVersion"=w668, "ClassDescription"=w677, "ClassProviderName"=w667, "ClassTemplateUsed"=w666) -> (w678:T10)
        n303 = call <resource>:"GDSLvClass_StoreClassType.vi"("Class Refnum In"=w661, "ClassSettings"=w678, "error in (no error)"=w669) -> ("error out"=w674:errorcluster)  [unwired: 15 in, 1 out]
      }
      frame "RemoveObjectRef_And_SaveFiles" {
        w700 = i32[] [1040, 1035] ("codes")
        n304 = Unbundle By Name(w716) -> ("BaseClass"=w708:refnum<vi>, "BaseObjectRef"=w714:path)
        n305 = Unbundle By Name(w716) -> ("ClassVIs"=w713:refnum<vi>[], "BaseAttrRef"=w711:refnum<vi>, "BaseClassAttrRef"=w710:refnum<vi>, "KernelRef"=w709:refnum<vi>)
        n306 = Build Array (concatenate)(w713, w711, w710, w709) -> (w712:refnum<vi>[])
        n307 = for {
          tunnel: w712 -> [w749] mode=indexing
          shift-right: [w750] -> w707
          shift-left: w717 -> [w751]
          n308 = Not A Number/Path/Refnum?(number/path/refnum=w749) -> (NaN/Path/Refnum?=w748:bool)
          n309 = case shown="True" w748 {
            tunnel: w751 -> [w756 w758]
            tunnel: [w754 w758] -> w750
            tunnel: w749 -> [w752 _]
            frame False {
              n310 = call <resource>:"Scripting_SaveVi.vi"("ForceResaving(False)"=FALSE, "error in (no error)"=w756, "VIRefToSaveIn"=w752) -> ("error out"=w755:errorcluster, "VIRefToSaveOut"=w757:refnum<vi>)  [unwired: 7 in]
              n311 = Close Reference(reference=w757, error in (no error)=w755) -> (error out=w754:errorcluster)
            }
            frame True {
            }
          }
        }
        n312 = invoke class="LVClassLibrary" method="Save"(reference=w708, error in=w707) -> (reference out=w705:refnum<vi>, error out=w706:errorcluster)  [unwired: 2 in, 2 out]
        n313 = case shown="False" w699 {
          tunnel: w714 -> [w728 _]
          tunnel: w706 -> [w724 w747]
          tunnel: w705 -> [w723 w746]
          tunnel: [w722 w746] -> w704
          tunnel: [w721 w747] -> w703
          tunnel: w700 -> [w720 _]
          frame False {
            n314 = property class="LVClassLibrary"(reference=w723, error in=w724) -> (reference out=w722:refnum<vi>, error out=w727:errorcluster, "Children[]"=w729:refnum<vi>[])
            n315 = call <resource>:"GDSError_ClearError.vi"("codes"=w720, "error in (no error)"=w727) -> ("error out"=w726:errorcluster)  [unwired: 16 in, 1 out]
            n316 = for {
              tunnel: w729 -> [w739] mode=indexing
              tunnel: w728 -> [w737]
              shift-right: [w731] -> w725
              shift-left: w726 -> [w733]
              n317 = property class="ProjectItem"(reference=w739, error in=w733) -> (reference out=w735:refnum<vi>, error out=w734:errorcluster, "Path"=w738:path)
              n318 = Equal?(x=w737, y=w738) -> (x = y?=w736:bool)
              n319 = case shown="True" w736 {
                tunnel: w735 -> [w740 w745]
                tunnel: [w741 w744] -> w732
                tunnel: w734 -> [w741 w742]
                tunnel: [w740 w743] -> w730
                frame False {
                }
                frame True {
                  n320 = invoke class="ProjectItem" method="Delete"(reference=w745, error in=w742) -> (reference out=w743:refnum<vi>, error out=w744:errorcluster)  [unwired: 1 in, 1 out]
                }
              }
              n321 = Close Reference(reference=w730, error in (no error)=w732) -> (error out=w731:errorcluster)
            }
            n322 = call <resource>:"GDSError_ClearError.vi"("codes"=w720, "error in (no error)"=w725) -> ("error out"=w721:errorcluster)  [unwired: 16 in, 1 out]
          }
          frame True {
          }
        }
        n323 = call <resource>:"GDSLvClass_SaveEverythingInClass.vi"("ClassRefIn"=w704, "error in"=w703) -> ("error out"=w702:errorcluster)  [unwired: 16 in, 1 out]
        n324 = call <resource>:"GDSError_ClearError.vi"("codes"=w700, "error in (no error)"=w702) -> ("error out"=w701:errorcluster)  [unwired: 16 in, 1 out]
        n325 = case shown="False" w699 {
          tunnel: w714 -> [w719 _]
          tunnel: w701 -> [w718 _]
          frame False {
            n326 = Delete(path (use dialog)=w719, error in=w718) -> ()  [unwired: 3 in, 3 out]
          }
          frame True {
          }
        }
      }
      frame "UpdateAllDerivedClasses" {
        n327 = case shown="False" w759 {
          tunnel: w762 -> [w767 w768]
          tunnel: [w766 w768] -> w761
          tunnel: w760 -> [w765 _]
          frame False {
            n328 = call <resource>:"Scripting_UpdateDerivedClasses.vi"("ClassRef"=w765, "error in (no error)"=w767) -> ("error out"=w766:errorcluster)  [unwired: 17 in]
          }
          frame True {
          }
        }
      }
      frame "CloseReferences", "Error" {
        n329 = call <resource>:"GDSError_LogErrorInformation.vi"("State"=w771, "LocalVariableData"=w770, "error in (no error)"=w772) -> ()  [unwired: 16 in, 1 out]
        n330 = Unbundle By Name(w770) -> ("NewBaseClass"=w776:refnum<vi>, "SubTemplateClass"=w774:refnum<vi>, "BaseTemplateClass"=w773:refnum<vi>, "App"=w769:refnum<vi>)
        n331 = Close Reference(reference=w774) -> ()  [unwired: 1 in, 1 out]
        n332 = Close Reference(reference=w773) -> ()  [unwired: 1 in, 1 out]
        n333 = Close Reference(reference=w776) -> ()  [unwired: 1 in, 1 out]
        n334 = Close Reference(reference=w769) -> ()  [unwired: 1 in, 1 out]
      }
    }
    n335 = Equal?(x=w30, y="Exit") -> (x = y?=w33:bool)
    n336 = Select(t="Error", s=w29, f=w30) -> (s? t:f=w34:string)
  }
  "error out" <- w14
  n337 = for {
    tunnel: w4 -> [w778] mode=indexing
    tunnel: w6 -> [w777] mode=indexing
    tunnel: w7 -> [_]
    n338 = Set Permissions(7:w777, 11:w778) -> ()  [unwired: 3 in, 2 out]
  }
